vi "Data Acquisition Testing.vi"(7 "write buffer":string, 8 "error in (no error)":errorcluster, 10 "stop":bool, 11 "VISA resource name":refnum<visa-resource-name>) -> (0 "error out":errorcluster, 5 "read buffer":string)   [LabVIEW 2024]
doc: "Test the write and read time of the connected instrument. Returns the average response time."
uses:
  <vilib>/Analysis/baseanly.llb/Mean (DBL).vi
  <vilib>/Analysis/NI_AALBase.lvlib
panel:
  out "error":i32
  out "mean":dbl format="%0.6f"
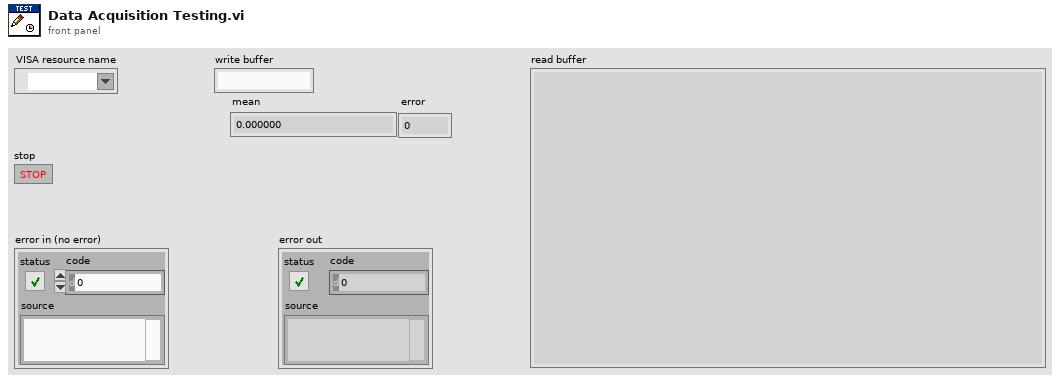
[diagram p1: front panel]
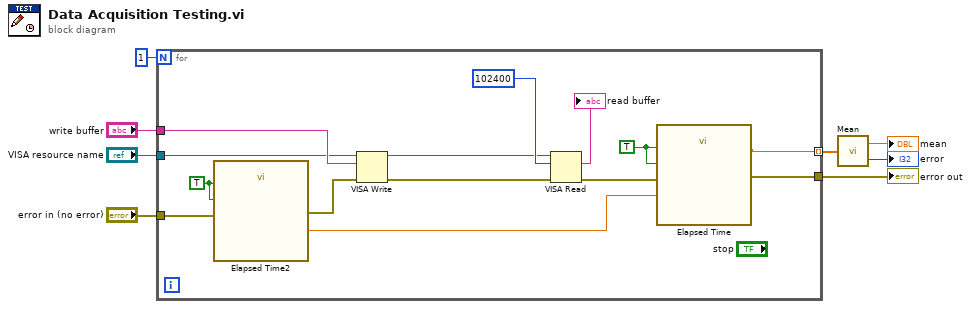
[diagram p0: block diagram]
diagram:
  n1 = for {
    N: 1 -> [_]
    tunnel: [w18] -> w8
    tunnel: "VISA resource name" -> [w13]
    tunnel: "write buffer" -> [w21]
    tunnel: "error in (no error)" -> [w16]
    tunnel: [w11] -> w4 mode=indexing
    w12 = TRUE ("Reset")
    w17 = TRUE ("Reset")
    n2 = call "Elapsed Time2"("Reset"=w12, "Auto Reset"=w12, "error in (no error)"=w16) -> ("Get Start Time (s)"=w14:dbl, "error out"=w15:errorcluster)  [unwired: 9 in, 6 out]
    n3 = VISA Write(VISA resource name=w13, write buffer=w21, error in (no error)=w15) -> (VISA resource name out=w9:refnum<visa-resource-name>, error out=w10:errorcluster)  [unwired: 1 out]
    n4 = VISA Read(VISA resource name=w9, byte count=u32 102400, error in (no error)=w10) -> (read buffer=→"read buffer":string, error out=w19:errorcluster)  [unwired: 2 out]
    n5 = call "Elapsed Time"("Reset"=w17, "Auto Reset"=w17, "error in (no error)"=w19, "Set Start Time (s)"=w14) -> ("Elapsed Time (s)"=w11:dbl, "error out"=w18:errorcluster)  [unwired: 8 in, 6 out]
  }
  "error out" <- w8
  n6 = call-poly <vilib>:"Mean.vi"("X"=w4) -> ("mean"=→"mean":dbl, "error"=→"error":i32)
